vi "Configure AM Internal [AM].vi"(7 "modulation waveform (Sine)":i32(ring)=1 items=["Sine"=1, "Square"=2, "Triangle"=3, "Ramp Up"=4, "Ramp Down"=5], 8 "error in (no error)":errorcluster, 9 "modulation frequency (1000 Hz)":dbl[unit]=1000.0 format="%^.2e", 10 "modulation depth (0.00 %)":dbl format="%.3f", 11 "CS++Fgen in":refnum<class "CS++Fgen.lvclass">) -> (0 "error out":errorcluster, 3 "CS++Fgen out":refnum<class "CS++Fgen.lvclass">)   [LabVIEW 2015, in "CS++Fgen.lvlib" / "CS++Fgen.lvclass"]
doc: "This VI configures the properties that control the function generator's internal amplitude modulation source. These properties are the modulation depth, waveform, and frequency.\n\nNotes:\n\n(1) This VI is part of the IviFgenModulateAM [AM] extension group."
uses:
  CS++Fgen.lvclass
  CSPP_Core/Classes/CS++ProcessVariables/ProcessVariable/PV.lvclass
  PV-Enum.ctl
  CS++Fgen.lvclass/CS++Fgen.ctl
  CSPP_Core/Classes/CS++ProcessVariables/ProcessVariable/PV.lvclass/PV.ctl
  CSPP_Core/Classes/CS++ProcessVariables/ProcessVariable/Write Data.vi
  CSPP_Core/Classes/CS++ProcessVariables/ProcessVariable/Write Timestamp.vi
  CSPP_Core/Classes/CS++ProcessVariables/ProcessVariable/Write Quality.vi
  CSPP_Core/Classes/CS++ProcessVariables/ProcessVariable/Write status.vi
  CSPP_Core/Classes/CS++ProcessVariables/PVConnection/PVConnection.lvclass
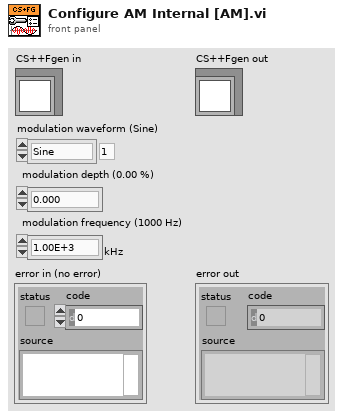
[diagram p1: front panel]
types:
  T1 = typedef "CS++Fgen.lvlib/CS++Fgen.lvclass/PV-Enum.ctl" = enum16{"AM-ModulationDepth", "AM-ModulationFrequency", "FM-ModulationFrequency", "FP-PeakDeviation", "SampleRate", "TriggerRate", "AM-ModulationWaveform", "FM-ModulationWaveform", "OutputMode", "ReferenceClockSource", "SampleClockSource", "SampleClockOutputEnabled"}
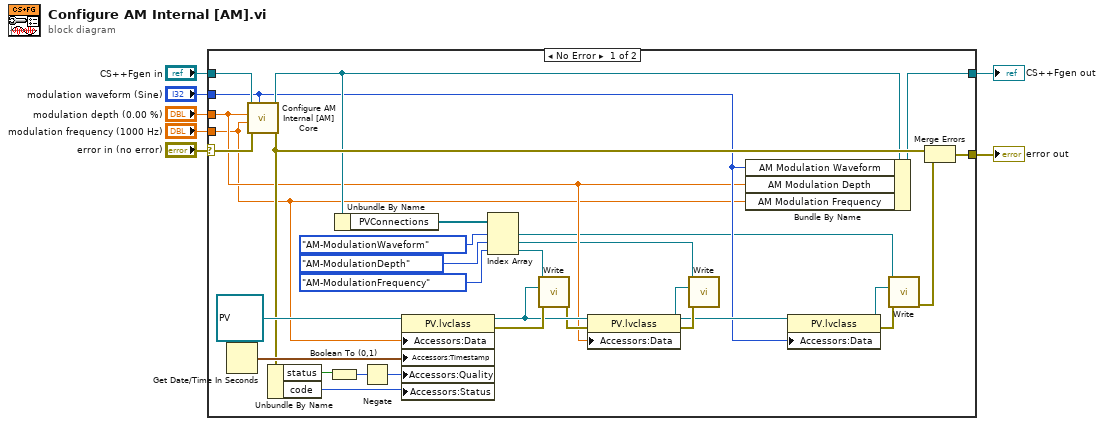
[diagram p0: block diagram]
diagram:
  n1 = case shown="No Error" "error in (no error)" {
    selector: "error in (no error)" -> [w36 w39]
    tunnel: [w18 w39] -> w6
    tunnel: [w26 w38] -> w4
    tunnel: "CS++Fgen in" -> [w37 w38]
    tunnel: "modulation waveform (Sine)" -> [w16 _]
    tunnel: "modulation depth (0.00 %)" -> [w15 _]
    tunnel: "modulation frequency (1000 Hz)" -> [w14 _]
    frame No Error {
      n2 = Get Date/Time In Seconds() -> (seconds since 1Jan1904=w35:timestamp)
      n3 = call-dynamic "Configure AM Internal [AM] Core.vi"("modulation waveform (Sine)"=w16, "error in (no error)"=w36, "modulation frequency (1000 Hz)"=w14, "modulation depth (0.00 %)"=w15, "CS++Fgen in"=w37) -> ("error out"=w28:errorcluster, "CS++Fgen out"=w27:refnum<class "CS++Fgen.lvclass">)  [unwired: 5 in]
      n4 = Unbundle By Name(w28) -> ("status"=w32:bool, "code"=w30:i32)
      n5 = Boolean To (0,1)(Boolean=w32) -> (0, 1=w31:i16)
      n6 = Unbundle By Name(w27) -> ("PVConnections"=w20:refnum<class "PVConnection.lvclass">[])
      n7 = Negate(x=w31) -> (-x=w29:i16)
      n8 = property class="PV.lvclass"(reference=refnum<class "PV.lvclass"> refnum ("PV"), "Accessors:Data"=w14, "Accessors:Timestamp"=w35, "Accessors:Quality"=w29, "Accessors:Status"=w30) -> (reference out=w24:refnum<class "PV.lvclass">, error out=w33:errorcluster)  [unwired: 1 in]
      n9 = Index Array(array=w20, index #1=PV-Enum."AM-ModulationWaveform" ("PV-Enum"), index #2=PV-Enum."AM-ModulationDepth" ("PV-Enum"), index #3=PV-Enum."AM-ModulationFrequency" ("PV-Enum")) -> (element #1=w8:refnum<class "PVConnection.lvclass">, element #2=w9:refnum<class "PVConnection.lvclass">, element #3=w12:refnum<class "PVConnection.lvclass">)
      n10 = call "Write.vi"("error in (no error)"=w33, "PV"=w24, "PVConnection in"=w12) -> ("error out"=w23:errorcluster)  [unwired: 7 in, 1 out]
      n11 = property class="PV.lvclass"(reference=w24, error in=w23, "Accessors:Data"=w15) -> (reference out=w19:refnum<class "PV.lvclass">, error out=w25:errorcluster)
      n12 = call "Write.vi"("error in (no error)"=w25, "PV"=w19, "PVConnection in"=w9) -> ()  [unwired: 7 in, 2 out]
      n13 = Bundle By Name(cluster=w27, "AM Modulation Waveform"=w16, "AM Modulation Depth"=w15, "AM Modulation Frequency"=w14) -> (w26:refnum<class "CS++Fgen.lvclass">)
      n14 = property class="PV.lvclass"(reference=w19, "Accessors:Data"=w16) -> (reference out=w21:refnum<class "PV.lvclass">, error out=w22:errorcluster)  [unwired: 1 in]
      n15 = call "Write.vi"("error in (no error)"=w22, "PV"=w21, "PVConnection in"=w8) -> ("error out"=w17:errorcluster)  [unwired: 7 in, 1 out]
      n16 = Merge Errors(w28, w17) -> (w18:errorcluster)
    }
    frame Error {
    }
  }
  "error out" <- w6
  "CS++Fgen out" <- w4
